vi "Untitled 2.vi"() -> ()   [LabVIEW 2014]
uses:
  <instrlib>/niHWS/nihws.llb/niHWS Open File Permissions ID.ctl
  <instrlib>/niHWS/nihws.llb/niHWS Write Analog DBL.vi
  <resource>/objmgr/daqmx.rc
  <instrlib>/niHWS/nihws.llb/niHWS Write Digital 2D U16.vi
  <vilib>/vision/NI_Vision_Development_Module.lvlib
  <instrlib>/niHWS/nihws.llb/niHWS Write Analog WDT.vi
  <vilib>/DAQmx/read.llb/DAQmx Read (Analog Wfm 1Chan NSamp).vi
  <vilib>/Analysis/NI_AALBase.lvlib
  <vilib>/Analysis/baseanly.llb/Mean (DBL).vi
  <vilib>/vision/Image Controls.llb/IMAQ Image.ctl
  <resource>/objmgr/IMAQImage.rc
  <vilib>/Utility/error.llb/DialogType.ctl
panel:
  in  "stop":bool
  out "Actual Fps":dbl
  out "Rec Time":dbl
  in  "Final res.":dbl=512.0
  out "Reported Fps":dbl caption="Frame Rate"
  out "Captured Frames":u32 caption="Image Number"
  out "Image Dst Out":T1
  out "Numeric":i32
  out "Photodiode display":waveform(dbl)(graph)
  out "Raw Image":T1(plugin-control)
  in  "Magnify":bool
  in  "Pixel Thr":dbl=4095.0
  in  "PseudoColor":bool
  in  "Analyze":bool
  in  "Recording Path":path
  out "file handle out":u32
  out "PPhocus?":bool
  out "Ephys Rate":dbl=1000.0
  in  "Rec":bool=TRUE
  out "Recording":bool
  out "Setup":i32
types:
  T1 = typedef "IMAQ Image.ctl" = refnum<image>
  T2 = typedef "niHWS Open File Permissions ID.ctl" = enum32{"Read Only", "Read/Write Existing", "Read/Write/Create New", "Read/Write/Create New Always"}
  T3 = enum32{"Average", "Min", "Max", "Clear  if < ", "Clear  if < or =", "Clear  if =", "Clear  if > or =", "Clear  if >"}
  T4 = enum32{"Gray", "Binary", "Gradient", "Rainbow", "Temperature"}
  T5 = enum32{"Invalid", "Standard", "Closed", "Hidden", "Minimized", "Maximized"}
  T6 = cluster{"IMAQ Session Out":refnum<k11>, "New Image":T1, "error out":errorcluster, cluster{dbl, i32}[], "New Image":T1}
  T7 = typedef "Image Type" = u32
  T8 = cluster{"IMAQ Session Out":refnum<k11>, "Image Out":T1, "error out":errorcluster, cluster{dbl, i32}[], "New Image":T1}
  T9 = typedef "DialogType.ctl" = u16
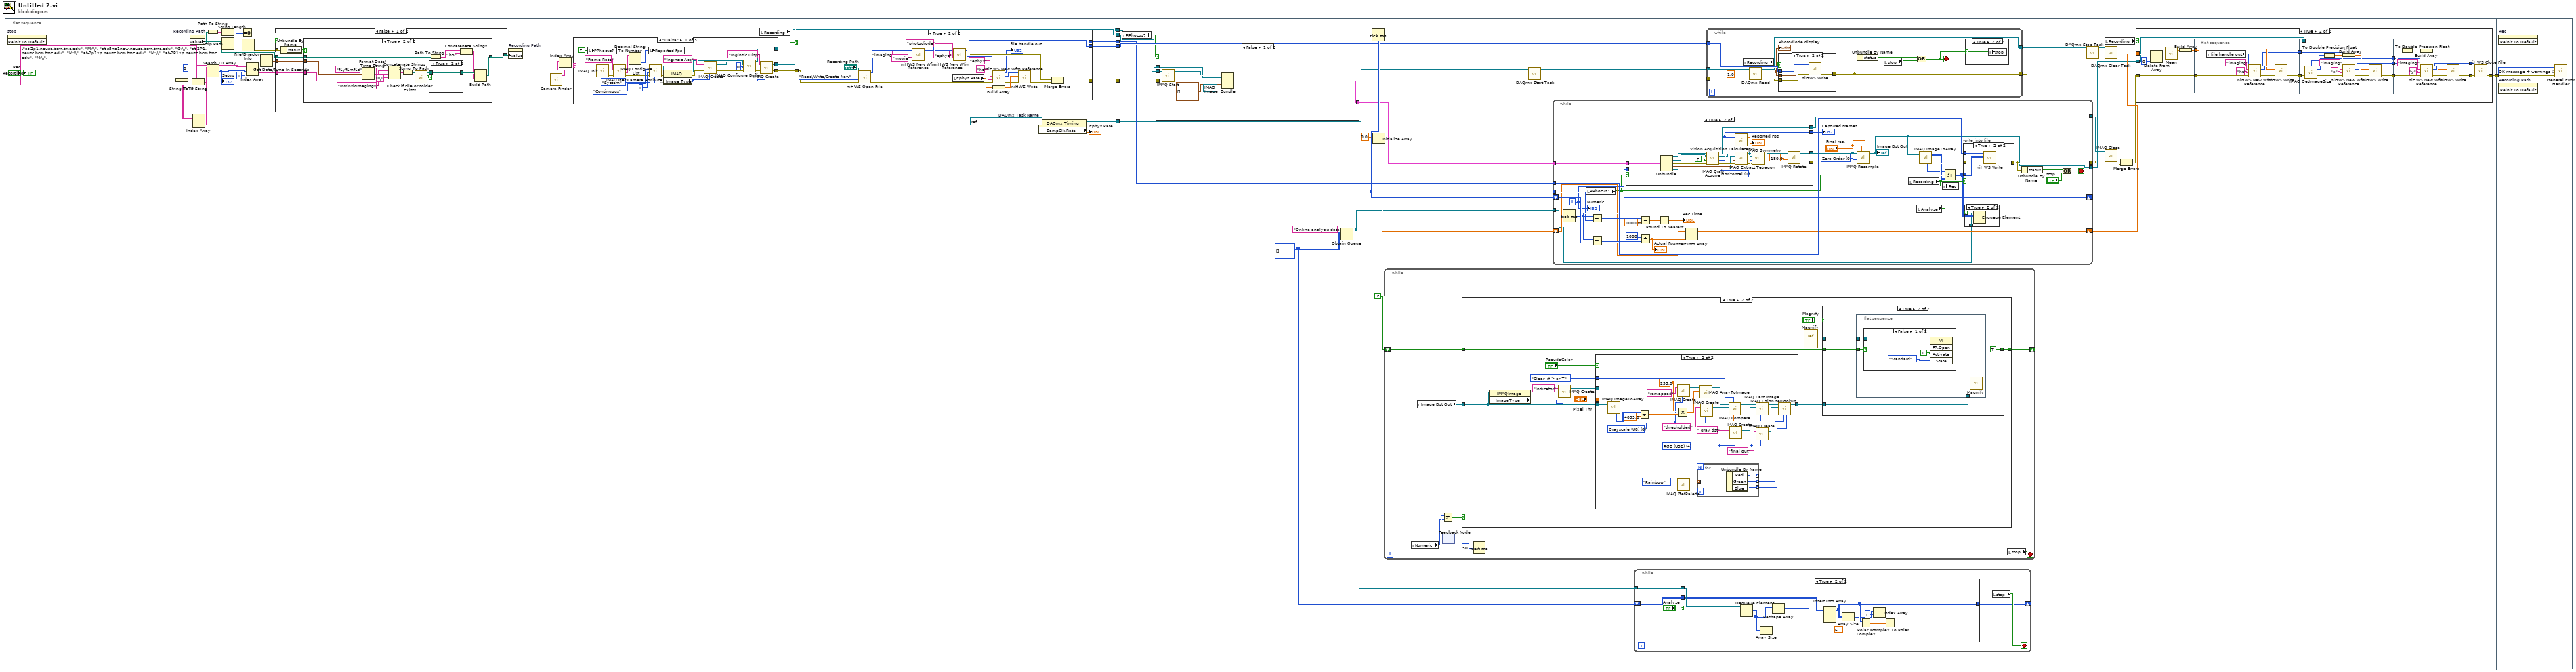
[diagram p0: block diagram]
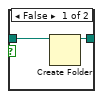
[diagram p3: hidden frame]
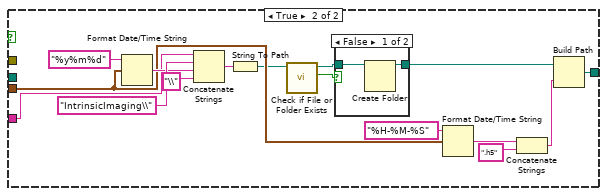
[diagram p4: hidden frame]
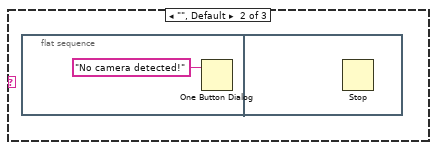
[diagram p6: hidden frame]
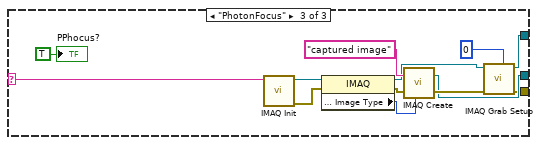
[diagram p7: hidden frame]
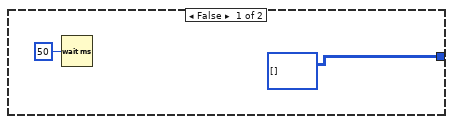
[diagram p9: hidden frame]
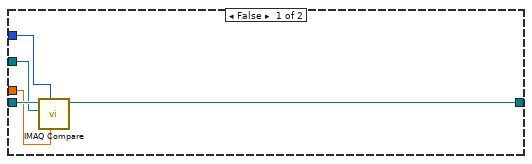
[diagram p11: hidden frame]
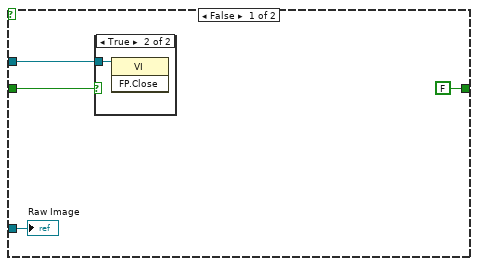
[diagram p12: hidden frame]
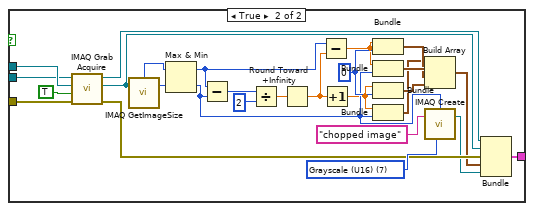
[diagram p15: hidden frame]
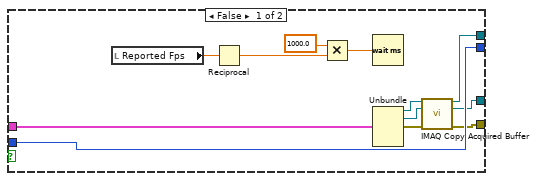
[diagram p20: hidden frame]
diagram:
  n1 = flat-sequence {
    tunnel: [w81] -> w7
    tunnel: [w80] -> w6
    tunnel: [w72] -> w5
    tunnel: [w76] -> w4
    tunnel: [w78] -> w3
    tunnel: [w73] -> w2
    tunnel: w7 -> [w169]
    tunnel: w6 -> [w170]
    tunnel: [w168] -> w1
    tunnel: w5 -> [w158]
    tunnel: w4 -> [w159]
    tunnel: w3 -> [w160]
    tunnel: w2 -> [w150]
    tunnel: w1 -> [w439]
    frame #0 {
      w9 = string[][] [["at-2p1.neusc.bcm.tmc.edu", "M:\\"], ["at-s5no1new.neusc.bcm.tmc.edu", "G:\\"], ["at-2P1.neusc.bcm.tmc.edu", "M:\\"], ["at-2p1xp.neusc.bcm.tmc.edu", "M:\\"], ["at-2P1xp.neusc.bcm.tmc.edu", "M:\\"]]
      n2 = invoke on="stop" class="Bool (strict)" method="Reinit To Default"() -> ()  [unwired: 3 in, 3 out]
      n3 = String To IP() -> (0:w15:u32)  [unwired: 1 in]
      n4 = property on="Recording Path" class="Path"() -> ("Value"=w18:path)  [unwired: 2 in, 2 out]
      n5 = IP To String(2:w15) -> (0:w10:string)  [unwired: 1 in]
      n6 = Index Array(array=w9, index (col)=0 ("disabled index (col)")) -> (element=w13:string[])  [unwired: 1 in]
      n7 = Path To String(path=w18) -> (string=w23:string)
      n8 = Search 1D Array(1D array=w13, element=w10) -> (index of element=w11:i32)  [unwired: 1 in]
      "Setup" <- w11
      n9 = String Length(string=w23) -> (length=w22:i32)
      n10 = Strip Path(path=w18) -> (stripped path=w17:path)  [unwired: 1 out]
      n11 = Equal To 0?(x=w22) -> (x = 0?=w21:bool)
      n12 = File/Directory Info(path=w17) -> (error out=w16:errorcluster)  [unwired: 1 in, 6 out]
      n13 = Index Array(array=w9, index (row)=w11, index (col)=1 ("disabled index (col)")) -> (element=w8:string)
      n14 = Get Date/Time In Seconds() -> (seconds since 1Jan1904=w24:timestamp)
      n15 = case shown="False" w21 {
        tunnel: w24 -> [w28 w57]
        tunnel: w18 -> [w29 _]
        tunnel: [w30 w55] -> w20
        tunnel: w16 -> [w26 _]
        tunnel: w8 -> [w25 w51]
        frame False {
          n16 = Unbundle By Name(w26) -> ("status"=w27:bool)
          n17 = case shown="True" w27 {
            tunnel: [w31 w38] -> w30
            tunnel: w29 -> [w31 w37]
            tunnel: w28 -> [_ w33]
            tunnel: w25 -> [_ w32]
            frame False {
            }
            frame True {
              n18 = Format Date/Time String(time format string (%c)="%y%m%d", seconds (now)=w33) -> (date/time string=w42:string)  [unwired: 1 in]
              n19 = Concatenate Strings(w32, "IntrinsicImaging\\", w42, "\\") -> (w41:string)
              n20 = String To Path(string=w41) -> (path=w47:path)
              n21 = call <vilib>:"Check if File or Folder Exists.vi"("path"=w47) -> ("file or folder exists?"=w45:bool, "dup path"=w44:path)  [unwired: 8 in, 1 out]
              n22 = case shown="True" w45 {
                tunnel: [w49 w50] -> w46
                tunnel: w44 -> [w48 w50]
                frame False {
                  n23 = Create Folder(path (use dialog)=w48) -> (created path=w49:path)  [unwired: 2 in, 2 out]
                }
                frame True {
                }
              }
              n24 = Path To String(path=w37) -> (string=w34:string)
              n25 = Concatenate Strings(w34, ".h5" ("string")) -> (w35:string)
              n26 = Build Path(base path=w46, name or relative path=w35) -> (appended path=w38:path)
            }
          }
        }
        frame True {
          n27 = Format Date/Time String(time format string (%c)="%y%m%d", seconds (now)=w57) -> (date/time string=w63:string)  [unwired: 1 in]
          n28 = Concatenate Strings(w51, "IntrinsicImaging\\", w63, "\\") -> (w64:string)
          n29 = String To Path(string=w64) -> (path=w56:path)
          n30 = call <vilib>:"Check if File or Folder Exists.vi"("path"=w56) -> ("file or folder exists?"=w60:bool, "dup path"=w61:path)  [unwired: 8 in, 1 out]
          n31 = case shown="False" w60 {
            tunnel: [w68 w69] -> w59
            tunnel: w61 -> [w67 w69]
            frame False {
              n32 = Create Folder(path (use dialog)=w67) -> (created path=w68:path)  [unwired: 2 in, 2 out]
            }
            frame True {
            }
          }
          n33 = Format Date/Time String(time format string (%c)="%H-%M-%S", seconds (now)=w57) -> (date/time string=w54:string)  [unwired: 1 in]
          n34 = Concatenate Strings(w54, ".h5" ("string")) -> (w52:string)
          n35 = Build Path(base path=w59, name or relative path=w52) -> (appended path=w55:path)
        }
      }
      n36 = property on="Recording Path" class="Path"("Value"=w20) -> ()  [unwired: 2 in, 2 out]
      "Recording" <- "Rec"
    }
    frame #1 {
      w75 = refnum<k21> "Photodiode Intrinsic Imaging"  # DAQmx Task Name
      n37 = call "Camera Finder.vi"() -> ("IMAQ Interfaces"=w70:string[])  [unwired: 11 in]
      n38 = Index Array(array=w70) -> (element=w71:string)  [unwired: 1 in]
      n39 = case shown="\"Dalsa\"" w71 {
        selector: w71 -> [w85 _ w110]
        tunnel: [w88 _ w113] -> w78
        tunnel: [w89 _ w112] -> w72
        tunnel: [w87 _ w111] -> w77
        frame "Dalsa" {
          n40 = local write "PPhocus?"(FALSE ("PPhocus?")) -> ()
          n41 = call <vilib>:"IMAQ Init.vi"("Interface Name"=w85) -> ("error out"=w90:errorcluster, "IMAQ Session Out"=w91:refnum<k11>)  [unwired: 9 in]
          n42 = call <vilib>:"IMAQ Get Camera Attribute.vi"("error in (no error)"=w90, "Camera Attribute"="Frame Rate", "IMAQ Session In"=w91) -> ("error out"=w82:errorcluster, "Attribute Value"=w84:string, "IMAQ Session Out"=w83:refnum<k11>)  [unwired: 4 in]
          n43 = Decimal String To Number(string=w84) -> (number=w86:i32)  [unwired: 2 in, 1 out]
          n44 = local write "Reported Fps"(w86) -> ()
          n45 = call <vilib>:"IMAQ Configure List.vi"("Memory Location"=enum16{"System", "Onboard"}."System", "error in (no error)"=w82, "Number of buffers"=u32 1, "Continuous?"=enum16{"One-Shot", "Continuous"}."Continuous" ("Continuous ?"), "IMAQ Session In"=w83) -> ("error out"=w99:errorcluster, "IMAQ Session Out"=w100:refnum<k11>)  [unwired: 5 in]
          n46 = property class="IMAQ"(reference=w100, error in=w99) -> (reference out=w98:refnum<k11>, error out=w97:errorcluster, "Image Parameters : Image Type"=w96:u32)
          n47 = call "IMAQ Create"("Image Name"="Inginsic Acq", "Image Type"=w96, "error in (no error)"=w97) -> ("New Image"=w93:T1, "error out"=w103:errorcluster)  [unwired: 2 in]
          n48 = call <vilib>:"IMAQ Configure Buffer.vi"("error in (no error)"=w103, "Buffer Number"=u32 0, "Image In"=w93, "IMAQ Session In"=w98) -> ("error out"=w95:errorcluster, "IMAQ Session Out"=w89:refnum<k11>)  [unwired: 6 in]
          n49 = call "IMAQ Create"("Image Name"="Inginsic Disp", "Image Type"=w96, "error in (no error)"=w95) -> ("New Image"=w88:T1, "error out"=w87:errorcluster)  [unwired: 2 in]
        }
        frame "", Default {
          n50 = flat-sequence {
            frame #0 {
              n51 = One Button Dialog(message="No camera detected!" ("error source (\" \")")) -> ()  [unwired: 1 in, 1 out]
            }
            frame #1 {
              n52 = Stop() -> ()  [unwired: 1 in]
            }
          }
        }
        frame "PhotonFocus" {
          n53 = call <vilib>:"IMAQ Init.vi"("Interface Name"=w110) -> ("error out"=w120:errorcluster, "IMAQ Session Out"=w119:refnum<k11>)  [unwired: 1 in, 8 out]
          n54 = property class="IMAQ"(reference=w119, error in=w120) -> (reference out=w114:refnum<k11>, error out=w117:errorcluster, "Image Parameters : Image Type"=w118:u32)
          n55 = call "IMAQ Create"("Image Name"="captured image", "Image Type"=w118, "error in (no error)"=w117) -> ("New Image"=w113:T1, "error out"=w115:errorcluster)  [unwired: 1 in, 1 out]
          n56 = call <vilib>:"IMAQ Grab Setup.vi"("Channel"=0, "error in (no error)"=w115, "IMAQ Session In"=w114) -> ("error out"=w111:errorcluster, "IMAQ Session Out"=w112:refnum<k11>)  [unwired: 7 out]
          "PPhocus?" <- TRUE ("PPhocus?")
        }
      }
      n57 = local read "Recording"() -> (w79:bool)
      n58 = case shown="True" w79 {
        tunnel: [_ w145] -> w81
        tunnel: [_ w125] -> w76
        tunnel: [_ w143] -> w80
        tunnel: w77 -> [_ w122]
        frame False {
        }
        frame True {
          n59 = call <instrlib>:"niHWS Open File.vi"("error in (no error)"=w122, "permissions (0:read only)"=niHWS_Open_File_Permissions_ID."Read/Write/Create New", "file path"="Recording Path") -> ("error out"=w140:errorcluster, "file handle"=w132:u32)  [unwired: 7 in]
          n60 = call <instrlib>:"niHWS New Wfm Reference.vi"("waveform name (empty)"="movie" ("format string"), "group name (empty)"="imaging", "file handle in"=w132) -> ("error out"=w128:errorcluster, "waveform reference"=w145:u32, "file handle out"=w129:u32)  [unwired: 6 in]
          n61 = local read "Ephys Rate"() -> (w123:dbl)
          n62 = call <instrlib>:"niHWS New Wfm Reference.vi"("error in (no error)"=w128, "waveform name (empty)"="photodiode", "group name (empty)"="ephys", "file handle in"=w129) -> ("error out"=w127:errorcluster, "waveform reference"=w143:u32, "file handle out"=w144:u32)  [unwired: 5 in]
          n63 = call <instrlib>:"niHWS New Wfm Reference.vi"("error in (no error)"=w140, "waveform name (empty)"="hz" ("group name (empty)"), "group name (empty)"="ephys", "file handle in"=w144) -> ("error out"=w135:errorcluster, "waveform reference"=w139:u32, "file handle out"=→"file handle out":u32)  [unwired: 5 in]
          n64 = Build Array(w123) -> (w136:dbl[])
          n65 = call-poly <instrlib>:"niHWS Write.vi"("error in (no error)"=w135, "data"=w136, "waveform reference in"=w139) -> ("error out"=w126:errorcluster)  [unwired: 7 in, 1 out]
          n66 = Merge Errors(w127, w126) -> (w125:errorcluster)
        }
      }
      n67 = property class="DAQmx Timing"(reference=w75) -> (reference out=w73:refnum<k21>, "SampClk.Rate"=→"Ephys Rate":dbl)  [unwired: 1 in, 1 out]
    }
    frame #2 {
      w146 = i32[][] []
      n68 = local read "PPhocus?"() -> (w152:bool)
      n69 = case shown="False" w152 {
        tunnel: w160 -> [w265 w294]
        tunnel: w159 -> [w267 w293]
        tunnel: w158 -> [w268 w292]
        tunnel: [w269 w272] -> w151
        frame False {
          n70 = call <vilib>:"IMAQ Start.vi"("error in (no error)"=w267, "IMAQ Session In"=w268) -> ("error out"=w264:errorcluster, "IMAQ Session Out"=w266:refnum<k11>)  [unwired: 8 in]
          n71 = Bundle("IMAQ Session Out"=w266, "New Image"=w265, "error out"=w264, cluster{dbl, i32}[] [], "New Image"=T1 refnum) -> (w269:T6)  [unwired: 1 in]
        }
        frame True {
          w288 = 0
          w295 = T7 7 items=["Grayscale (U8)", "Grayscale (I16)", "Grayscale (SGL)", "Complex (CSG)", "RGB (U32)", "HSL (U32)", "RGB (U64)", "Grayscale (U16)"] ("Image Type")
          n72 = call <vilib>:"IMAQ Grab Acquire.vi"("error in (no error)"=w293, "Immediate?"=TRUE, "Image In"=w294, "IMAQ Session In"=w292) -> ("error out"=w273:errorcluster, "Image Out"=w274:T1, "IMAQ Session Out"=w275:refnum<k11>)  [unwired: 5 out]
          n73 = call "IMAQ GetImageSize"("Image"=w274) -> ("Y Resolution"=w289:i32, "X Resolution"=w290:i32)  [unwired: 3 in, 1 out]
          n74 = Max & Min(x=w290, y=w289) -> (max(x,y)=w281:i32, min(x,y)=w287:i32)
          n75 = Subtract(x=w281, y=w287) -> (x-y=w286:i32)
          n76 = Divide(x=w286, y=2) -> (x/y=w284:dbl)
          n77 = Round Toward +Infinity(x=w284) -> (ceil(x): smallest int >= x=w282:dbl)
          n78 = Subtract(x=w281, y=w282) -> (x-y=w280:dbl)
          n79 = Increment(x=w282) -> (x+1=w283:dbl)
          n80 = Bundle(w280, w288) -> (w278:cluster{dbl, i32})  [unwired: 1 in]
          n81 = Bundle(w280, w287) -> (w279:cluster{dbl, i32})  [unwired: 1 in]
          n82 = Bundle(w283, w288) -> (w277:cluster{dbl, i32})  [unwired: 1 in]
          n83 = Bundle(w283, w287) -> (w276:cluster{dbl, i32})  [unwired: 1 in]
          n84 = Build Array(w276, w279, w278, w277) -> (w271:cluster{dbl, i32}[])
          n85 = call "IMAQ Create"("Border Size"=w287, "Image Name"="chopped image", "Image Type"=w295) -> ("New Image"=w270:T1)  [unwired: 1 in, 2 out]
          n86 = Bundle("IMAQ Session Out"=w275, "Image Out"=w274, "error out"=w273, w271, "New Image"=w270) -> (w272:T8)  [unwired: 1 in]
        }
      }
      n87 = Obtain Queue(name (unnamed)="Online analysis data", element data type=w146) -> (queue out=w147:refnum<queue>)  [unwired: 3 in, 2 out]
      n88 = Tick Count (ms)() -> (millisecond timer value=w175:u32)
      n89 = Initialize Array(0.0 ("element")) -> (w166:dbl[])  [unwired: 1 in]
      n90 = while {
        shift-right: [w197] -> _
        shift-left: FALSE -> [w196]
        stop <- w198 stop-if-true
        n91 = local read "Numeric"() -> (w192:i32)
        n92 = local read "Image Dst Out"() -> (w194:T1)
        n93 = feedback-in #1(w192) -> ()
        n94 = feedback #1() -> (w193:i32)  [unwired: 1 in]
        n95 = Not Equal?(x=w193, y=w192) -> (x != y?=w191:bool)
        n96 = case shown="True" w191 {
          tunnel: [w199 w209] -> w197
          tunnel: w196 -> [w199 w208]
          tunnel: w194 -> [_ w200]
          frame False {
          }
          frame True {
            n97 = property class="IMAQImage"(reference=w200) -> ("ImageType"=w201:i32)  [unwired: 1 in, 2 out]
            n98 = call "IMAQ Create"("Image Name"="Indicator", "Image Type"=w201) -> ("New Image"=w206:T1)  [unwired: 3 in, 1 out]
            n99 = case shown="True" "PseudoColor" {
              tunnel: w200 -> [w216 w231]
              tunnel: w206 -> [w215 _]
              tunnel: T3."Clear  if > or =" ("Operator") -> [w214 w226]
              tunnel: "Pixel Thr" -> [w213 _]
              tunnel: [w212 w220] -> w203
              frame False {
                n100 = call "IMAQ Compare"("Constant"=w213, "Operator"=w214, "Image Dst"=w215, "Image Src A"=w216) -> ("Image Dst Out"=w212:T1)  [unwired: 6 in, 1 out]
              }
              frame True {
                w219 = T7 0 items=["Grayscale (U8)", "Grayscale (I16)", "Grayscale (SGL)", "Complex (CSG)", "RGB (U32)", "HSL (U32)", "RGB (U64)", "Grayscale (U16)"] ("Image Type")
                w221 = 255.0 ("x")
                w218 = T7 4 items=["Grayscale (U8)", "Grayscale (I16)", "Grayscale (SGL)", "Complex (CSG)", "RGB (U32)", "HSL (U32)", "RGB (U64)", "Grayscale (U16)"] ("Image Type")
                n101 = call "IMAQ ImageToArray"("Image"=w231) -> ("Image Pixels (U16)"=w230:u16[][])  [unwired: 3 in, 4 out]
                n102 = Divide(x=w230, y=4095.0) -> (x/y=w233:dbl[][])
                n103 = Multiply(x=w221, y=w233) -> (x*y=w229:dbl[][])
                n104 = call "IMAQ Create"("Image Name"="remapped", "Image Type"=w219) -> ("New Image"=w227:T1)  [unwired: 3 in, 1 out]
                n105 = call "IMAQ GetPalette"("Palette Number (gray)"=T4."Rainbow") -> ("Color Palette"=w238:cluster{"Red":u8, "Green":u8, "Blue":u8}[])  [unwired: 4 in, 1 out]
                n106 = for {
                  tunnel: w238 -> [w246] mode=indexing
                  tunnel: [w245] -> w239 mode=indexing
                  tunnel: [w244] -> w240 mode=indexing
                  tunnel: [w243] -> w241 mode=indexing
                  n107 = Unbundle By Name(w246) -> ("Red"=w245:u8, "Green"=w244:u8, "Blue"=w243:u8)
                }
                n108 = call "IMAQ ArrayToImage"("Image Pixels (U8)"=w229, "Image"=w227) -> ("Image Out"=w222:T1)  [unwired: 8 in, 1 out]
                n109 = call "IMAQ Create"("Image Name"="thresholded", "Image Type"=w219) -> ("New Image"=w224:T1)  [unwired: 3 in, 1 out]
                n110 = call "IMAQ Compare"("Constant"=w221, "Operator"=w226, "Image Dst"=w224, "Image Src A"=w222) -> ("Image Dst Out"=w223:T1)  [unwired: 6 in, 1 out]
                n111 = call "IMAQ Create"("Image Name"=" gray dst", "Image Type"=w218) -> ("New Image"=w236:T1)  [unwired: 2 in, 2 out]
                n112 = call "IMAQ Cast Image"("Image Type"=w218, "Image Dst"=w236, "Image Src"=w223) -> ("Image Dst Out"=w234:T1)  [unwired: 7 in, 1 out]
                n113 = call "IMAQ Create"("Image Name"="final out", "Image Type"=w218) -> ("New Image"=w242:T1)  [unwired: 3 in, 1 out]
                n114 = call "IMAQ ColorUserLookup"("Blue or Luma or Val or Inten Lookup Table"=w241, "Green or Sat Lookup Table"=w240, "Red or Hue Lookup Table"=w239, "Image Dst"=w242, "Image Src"=w234) -> ("Image Dst Out"=w220:T1)  [unwired: 5 in, 1 out]
              }
            }
            n115 = vi-ref "Magnify.vi"() -> (w211:refnum<vi>)
            n116 = case shown="True" "Magnify" {
              tunnel: w211 -> [w250 w255]
              tunnel: [FALSE TRUE] -> w209
              tunnel: w208 -> [w249 w253]
              tunnel: w203 -> [w247 w252]
              frame False {
                n117 = case shown="True" w249 {
                  tunnel: w250 -> [_ w251]
                  frame False {
                  }
                  frame True {
                    n118 = invoke class="VI" method="FP.Close"(reference=w251) -> ()  [unwired: 2 in, 3 out]
                  }
                }
                "Raw Image" <- w247
              }
              frame True {
                n119 = flat-sequence {
                  tunnel: w255 -> [w257]
                  tunnel: w253 -> [w256]
                  tunnel: w252 -> [w261]
                  frame #0 {
                    n120 = case shown="False" w256 {
                      tunnel: w257 -> [w259 _]
                      frame False {
                        n121 = invoke class="VI" method="FP.Open"(reference=w259, "Activate"=TRUE ("Wait Until Done"), "State"=T5."Standard") -> ()  [unwired: 2 in, 5 out]
                      }
                      frame True {
                      }
                    }
                  }
                  frame #1 {
                    n122 = call "Magnify.vi"("Camera 2"=w261) -> ()  [unwired: 11 in]
                  }
                }
              }
            }
          }
        }
        n123 = Wait (ms)(milliseconds to wait=u32 50) -> ()  [unwired: 1 out]
        n124 = local read "stop"() -> (w198:bool)
      }
      n125 = call <vilib>:"DAQmx Start Task.vi"("task/channels in"=w150) -> ("task out"=w173:refnum<k21>, "error out"=w167:errorcluster)  [unwired: 13 in]
      n126 = while {
        tunnel: w169 -> [w399]
        shift-right: [w394] -> _
        shift-left: w175 -> [w398]
        tunnel: w175 -> [w393]
        shift-right: [w387] -> w164
        shift-left: w166 -> [w388]
        tunnel: [w383] -> w155
        tunnel: [w372] -> w163
        tunnel: [w368] -> w157
        tunnel: w151 -> [w374]
        tunnel: w147 -> [w366]
        i -> [w375]
        stop <- w384 stop-if-true
        w373 = u32 0 items=["Zero Order", "Bi-Linear", "Quadratic", "Cubic Spline"] ("Interpolation Type")
        n127 = Tick Count (ms)() -> (millisecond timer value=w394:u32)
        n128 = local read "PPhocus?"() -> (w371:bool)
        n129 = Subtract(x=w394, y=w393) -> (x-y=w392:u32)
        n130 = Subtract(x=w394, y=w398) -> (x-y=w397:u32)
        n131 = case shown="True" w371 {
          tunnel: [w408 w432] -> w372
          tunnel: [w407 w416] -> w379
          tunnel: [w406 w415] -> w378
          tunnel: [w413 w427] -> w376
          tunnel: w375 -> [w413 _]
          tunnel: w374 -> [w412 w426]
          frame False {
            n132 = local read "Reported Fps"() -> (w405:dbl)
            n133 = Reciprocal(x=w405) -> (1/x=w404:dbl)
            n134 = Multiply(x=1000.0, y=w404) -> (x*y=w402:dbl)
            n135 = Wait (ms)(milliseconds to wait=w402) -> ()  [unwired: 1 out]
            n136 = Unbundle(w412) -> ("IMAQ Session Out"=w411:refnum<k11>, "Image Out"=w410:T1, "error out"=w409:errorcluster)  [unwired: 2 out]
            n137 = call <vilib>:"IMAQ Copy Acquired Buffer.vi"("IMAQ Session In"=w411, "Image In"=w410, "error in (no error)"=w409) -> ("IMAQ Session Out"=w408:refnum<k11>, "Image Out"=w407:T1, "error out"=w406:errorcluster)  [unwired: 8 in, 2 out]
          }
          frame True {
            w431 = u32 0 items=["Horizontal", "Vertical", "Central", "1st Diagonal", "2nd Diagonal"] ("Type of Symmetry")
            n138 = Unbundle(w426) -> ("IMAQ Session Out"=w425:refnum<k11>, "Image Out"=w424:T1, "error out"=w423:errorcluster, w422:cluster{dbl, i32}[], "New Image"=w421:T1)
            n139 = call <vilib>:"IMAQ Grab Acquire.vi"("error in (no error)"=w423, "Immediate?"=FALSE, "Image In"=w424, "IMAQ Session In"=w425) -> ("error out"=w430:errorcluster, "Acquired Buffer Number"=w427:u32, "Image Out"=w420:T1, "IMAQ Session Out"=w432:refnum<k11>)  [unwired: 4 out]
            n140 = call <vilib>:"Vision Acquisition CalculateFPS.vi"("buffer number"=w427) -> ("acquired FPS"=→"Reported Fps":dbl)  [unwired: 2 out]
            n141 = call-poly "IMAQ Extract Tetragon"("error in (no error)"=w430, "Tetragon"=w422, "Image Dst"=w421, "Image Src"=w420) -> ("error out"=w429:errorcluster, "Image Dst Out"=w428:T1)  [unwired: 6 in]
            n142 = call "IMAQ Symmetry"("error in (no error)"=w429, "Type of Symmetry"=w431, "Image Dst"=w428, "Image Src"=w428) -> ("error out"=w417:errorcluster, "Image Dst Out"=w418:T1)  [unwired: 1 in]
            n143 = call "IMAQ Rotate"("error in (no error)"=w417, "Angle (degrees)"=sgl 180.0, "Image Src"=w418) -> ("error out"=w415:errorcluster, "Image Dst Out"=w416:T1)  [unwired: 7 in]
          }
        }
        "Captured Frames" <- w376
        n144 = Divide(x=w392, y=1000.0) -> (x/y=w391:dbl)
        n145 = Divide(x=u32 1000, y=w397) -> (x/y=w389:dbl)
        "Actual Fps" <- w389
        n146 = Round To Nearest(number=w391) -> (nearest integer value=→"Rec Time":dbl)
        n147 = Insert Into Array(array=w388, new element=w389) -> (w387:dbl[])  [unwired: 1 in]
        n148 = call "IMAQ Resample"("X Resolution"="Final res.", "Y Resolution"="Final res.", "error in (no error)"=w378, "Interpolation Type"=w373, "Image Dst"=w379, "Image Src"=w379) -> ("error out"=w377:errorcluster, "Image Dst Out"=w368:T1)  [unwired: 4 in]
        "Image Dst Out" <- w368
        n149 = local read "Recording"() -> (w380:bool)
        n150 = local read "Analyze"() -> (w365:bool)
        n151 = call "IMAQ ImageToArray"("error in (no error)"=w377, "Image"=w368) -> ("Image Pixels (U16)"=w369:u16[][], "error out"=w382:errorcluster, "Image Pixels (I16)"=w370:i16[][])  [unwired: 2 in, 2 out]
        n152 = local write "Rec"(w380) -> ()
        n153 = Select(t=w369, s=w371, f=w370) -> (s? t:f=w367:u16[][])
        n154 = case "write into file" shown="True" w380 {
          tunnel: w382 -> [w434 w437]
          tunnel: w367 -> [_ w438]
          tunnel: [w434 w436] -> w383
          tunnel: w399 -> [_ w435]
          frame False {
          }
          frame True {
            n155 = call-poly <instrlib>:"niHWS Write.vi"("error in (no error)"=w437, "data"=w438, "waveform reference in"=w435) -> ("error out"=w436:errorcluster)  [unwired: 7 in, 1 out]
          }
        }
        n156 = case shown="True" w365 {
          tunnel: w367 -> [_ w401]
          tunnel: w366 -> [_ w400]
          frame False {
          }
          frame True {
            n157 = Enqueue Element(queue=w400, element=w401) -> ()  [unwired: 2 in, 3 out]
          }
        }
        n158 = Unbundle By Name(w383) -> ("status"=w381:bool)
        n159 = Or(x=w381, y="stop") -> (x .or. y?=w384:bool)
        "Numeric" <- w375
      }
      n160 = while {
        tunnel: w147 -> [w178]
        shift-right: [w176] -> _
        shift-left: w146 -> [w177]
        stop <- w180 stop-if-true
        n161 = case shown="True" "Analyze" {
          tunnel: w178 -> [_ w190]
          tunnel: w177 -> [_ w187]
          tunnel: [i32[][] [] w185] -> w176
          frame False {
            n162 = Wait (ms)(milliseconds to wait=u32 50) -> ()  [unwired: 1 out]
          }
          frame True {
            (unwired) 6.283185307179586
            n163 = Dequeue Element(queue=w190) -> (element=w189:i32[][])  [unwired: 2 in, 3 out]
            n164 = Array Size(array=w189) -> ()  [unwired: 1 out]
            n165 = Reshape Array(w189) -> (w188:i32[])  [unwired: 1 in]
            n166 = Insert Into Array(array=w187, new element=w188) -> (w185:i32[][])  [unwired: 2 in]
            n167 = Array Size(array=w185) -> (size(s)=w184:i32[])
            n168 = Polar To Complex(2:w185) -> (0:w186:cdb[][])  [unwired: 1 in]
            n169 = Index Array(array=w184, index=1) -> ()  [unwired: 1 out]
            n170 = Complex To Polar(r * e^(i*theta)=w186) -> ()  [unwired: 2 out]
          }
        }
        n171 = local read "stop"() -> (w180:bool)
      }
      n172 = while {
        tunnel: w173 -> [w358]
        tunnel: w167 -> [w354]
        tunnel: w170 -> [w357]
        tunnel: [w351] -> w156
        tunnel: [w355] -> w174
        stop <- w347 stop-if-true
        n173 = local read "Recording"() -> (w352:bool)
        n174 = call-poly <vilib>:"DAQmx Read.vi"("task/channels in"=w358, "timeout"=-1.0, "error in"=w354) -> ("task out"=w355:refnum<k21>, "data"=w356:waveform(dbl), "error out"=w350:errorcluster)  [unwired: 10 in]
        "Photodiode display" <- w356
        n175 = case shown="True" w352 {
          tunnel: w356 -> [_ w361]
          tunnel: w357 -> [_ w364]
          tunnel: [w360 w363] -> w351
          tunnel: w350 -> [w360 w362]
          frame False {
          }
          frame True {
            n176 = call-poly <instrlib>:"niHWS Write.vi"("error in (no error)"=w362, "analog waveform"=w361, "waveform reference in"=w364) -> ("error out"=w363:errorcluster)  [unwired: 7 in, 1 out]
          }
        }
        n177 = Unbundle By Name(w351) -> ("status"=w348:bool)
        n178 = local read "stop"() -> (w353:bool)
        n179 = Or(x=w348, y=w353) -> (x .or. y?=w347:bool)
        n180 = case shown="True" w347 {
          selector: w347 -> [_ w359]
          frame False {
          }
          frame True {
            n181 = local write "stop"(w359) -> ()
          }
        }
      }
      n182 = call <vilib>:"DAQmx Stop Task.vi"("task/channels in"=w174, "error in"=w156) -> ("task out"=w171:refnum<k21>, "error out"=w172:errorcluster)  [unwired: 12 in]
      n183 = local read "Recording"() -> (w153:bool)
      n184 = call <vilib>:"DAQmx Clear Task.vi"("task in"=w171, "error in"=w172) -> ("error out"=w154:errorcluster)  [unwired: 13 in]
      n185 = call <vilib>:"IMAQ Close.vi"("error in (no error)"=w155, "IMAQ Session In"=w163) -> ("error out"=w162:errorcluster)  [unwired: 9 out]
      n186 = Merge Errors(w162, w154) -> (w161:errorcluster)
      n187 = case shown="True" w153 {
        tunnel: [w297 w312] -> w168
        tunnel: w164 -> [_ w311]
        tunnel: w161 -> [w297 w298]
        tunnel: w157 -> [_ w299]
        frame False {
        }
        frame True {
          n188 = Delete From Array(array=w311, index=0) -> (array with subset deleted=w309:dbl[])  [unwired: 1 in, 1 out]
          n189 = call-poly <vilib>:"Mean.vi"("X"=w309) -> ("mean"=w310:dbl)  [unwired: 1 out]
          n190 = Build Array(w310) -> (w305:dbl[])
          n191 = flat-sequence {
            tunnel: w305 -> [w316]
            tunnel: [w321] -> w307
            tunnel: [w315] -> w306
            tunnel: w298 -> [w314]
            tunnel: w307 -> [w323]
            tunnel: w306 -> [w332]
            tunnel: [w331] -> w304
            tunnel: [w329] -> w302
            tunnel: [w325] -> w300
            tunnel: w299 -> [w322]
            tunnel: w304 -> [w343]
            tunnel: [w342] -> w303
            tunnel: w302 -> [w341]
            tunnel: [w339] -> w301
            tunnel: w300 -> [w336]
            frame #0 {
              n192 = local read "file handle out"() -> (w313:u32)
              n193 = call <instrlib>:"niHWS New Wfm Reference.vi"("error in (no error)"=w314, "waveform name (empty)"="hz" ("group name (empty)"), "group name (empty)"="imaging", "file handle in"=w313) -> ("error out"=w317:errorcluster, "waveform reference"=w318:u32, "file handle out"=w315:u32)  [unwired: 5 in]
              n194 = call-poly <instrlib>:"niHWS Write.vi"("error in (no error)"=w317, "data"=w316, "waveform reference in"=w318) -> ("error out"=w321:errorcluster)  [unwired: 7 in, 1 out]
            }
            frame #1 {
              n195 = call "IMAQ GetImageSize"("Image"=w322, "error in (no error)"=w323) -> ("Y Resolution"=w325:i32, "X Resolution"=w326:i32, "error out"=w324:errorcluster)  [unwired: 2 in]
              n196 = To Double Precision Float(number=w326) -> (double precision float=w327:dbl)
              n197 = Build Array(w327) -> (w328:dbl[])
              n198 = call <instrlib>:"niHWS New Wfm Reference.vi"("error in (no error)"=w324, "waveform name (empty)"="x" ("group name (empty)"), "group name (empty)"="imaging", "file handle in"=w332) -> ("error out"=w330:errorcluster, "waveform reference"=w333:u32, "file handle out"=w331:u32)  [unwired: 5 in]
              n199 = call-poly <instrlib>:"niHWS Write.vi"("error in (no error)"=w330, "data"=w328, "waveform reference in"=w333) -> ("error out"=w329:errorcluster)  [unwired: 7 in, 1 out]
            }
            frame #2 {
              n200 = To Double Precision Float(number=w336) -> (double precision float=w337:dbl)
              n201 = Build Array(w337) -> (w338:dbl[])
              n202 = call <instrlib>:"niHWS New Wfm Reference.vi"("error in (no error)"=w341, "waveform name (empty)"="y" ("group name (empty)"), "group name (empty)"="imaging", "file handle in"=w343) -> ("error out"=w340:errorcluster, "waveform reference"=w346:u32, "file handle out"=w342:u32)  [unwired: 5 in]
              n203 = call-poly <instrlib>:"niHWS Write.vi"("error in (no error)"=w340, "data"=w338, "waveform reference in"=w346) -> ("error out"=w339:errorcluster)  [unwired: 7 in, 1 out]
            }
          }
          n204 = call <instrlib>:"niHWS Close File.vi"("error in (no error)"=w301, "file handle"=w303) -> ("error out"=w312:errorcluster)  [unwired: 9 in]
        }
      }
    }
    frame #3 {
      w440 = T9 3 items=["no dialog", "OK message", "continue or stop message", "OK message + warnings", "continue/stop + warnings"] ("type of dialog (OK msg:1)")
      n205 = invoke on="Rec" class="Bool (strict)" method="Reinit To Default"() -> ()  [unwired: 3 in, 3 out]
      n206 = invoke on="Recording Path" class="Path" method="Reinit To Default"() -> ()  [unwired: 3 in, 3 out]
      n207 = call <vilib>:"General Error Handler.vi"("type of dialog (OK msg:1)"=w440, "error in (no error)"=w439) -> ()  [unwired: 9 in, 5 out]
    }
  }
